vi "settings.vi"(8 "error in":errorcluster, 10 "Array":T1[](array[typedef]), 11 "notifier":refnum<notifier>) -> (0 "error out":errorcluster)   [LabVIEW 2015]
uses:
  Type Definitions/vars_settings.ctl
panel:
  in  "Cancel Button":bool
  in  "OK Button":bool
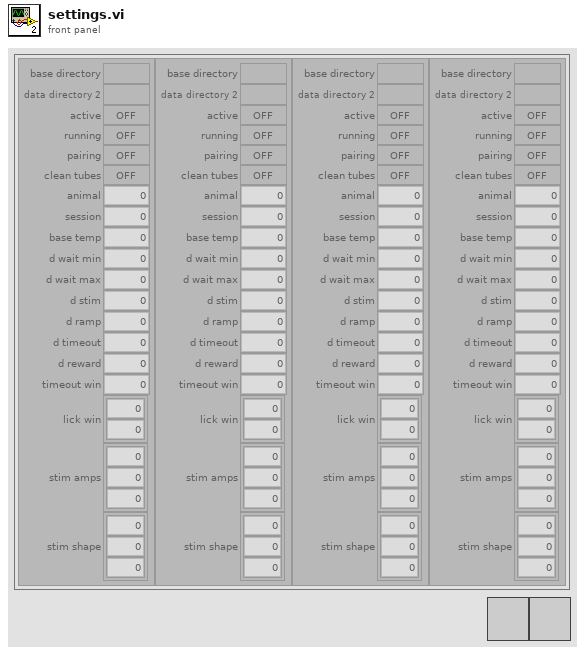
[diagram p1: front panel]
types:
  T1 = typedef "vars_settings.ctl" = cluster{"base directory":path, "data directory 2":path, "active":bool, "running":bool, "pairing":bool, "clean tubes":bool, "animal":u16, "session":u16, "base temp":sgl, "d wait min":u16, "d wait max":u16, "d stim":u16, "d ramp":u16, "d timeout":u16, "d reward":u16, "timeout win":u16, "lick win":i32[], "stim amps":dbl[], "stim shape":dbl[]}
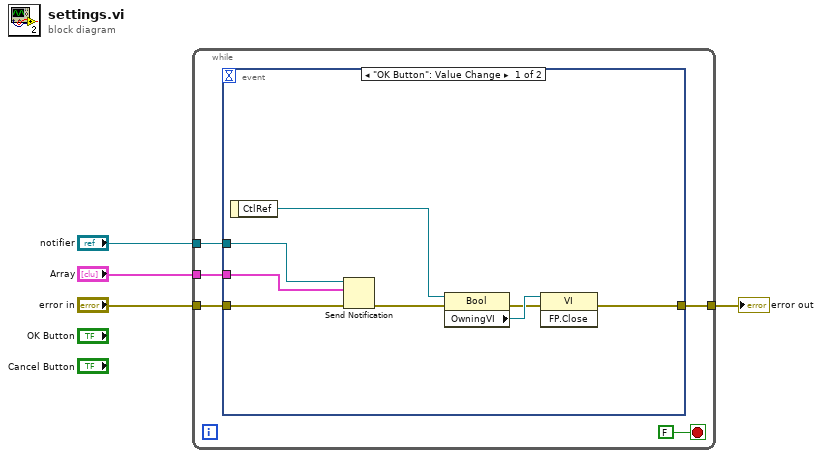
[diagram p0: block diagram]
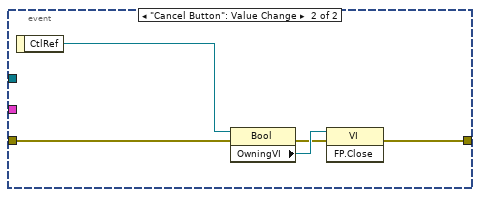
[diagram p2: hidden frame]
diagram:
  n1 = while {
    tunnel: "notifier" -> [w9]
    tunnel: "Array" -> [w8]
    tunnel: "error in" -> [w7]
    tunnel: [w6] -> w1
    stop <- FALSE stop-if-true
    n2 = event shown="[0] \"OK Button\": Value Change" {
      selector: _ -> [_ _]
      dyn-events: _ -> [_ _]
      timeout: _ -> [_ _]
      tunnel: w9 -> [w17 _]
      tunnel: w8 -> [w16 _]
      tunnel: w7 -> [w11 w18]
      tunnel: [w10 w19] -> w6
      event "OK Button": Value Change {
        n3 = event-data() -> ("CtlRef"=w15:refnum<vi>)  [unwired: 1 in]
        n4 = Send Notification(notification=w16, notifier=w17, error in (no error)=w11) -> (error out=w13:errorcluster)  [unwired: 1 out]
        n5 = property class="Bool"(reference=w15, error in=w13) -> (error out=w12:errorcluster, "OwningVI"=w14:refnum<vi>)  [unwired: 1 out]
        n6 = invoke class="VI" method="FP.Close"(reference=w14, error in=w12) -> (error out=w10:errorcluster)  [unwired: 1 in, 2 out]
      }
      event "Cancel Button": Value Change {
        n7 = event-data() -> ("CtlRef"=w22:refnum<vi>)  [unwired: 1 in]
        n8 = property class="Bool"(reference=w22, error in=w18) -> (error out=w20:errorcluster, "OwningVI"=w21:refnum<vi>)  [unwired: 1 out]
        n9 = invoke class="VI" method="FP.Close"(reference=w21, error in=w20) -> (error out=w19:errorcluster)  [unwired: 1 in, 2 out]
      }
    }
  }
  "error out" <- w1
